vi "Get SMO Name.vi"(8 "error in (no error)":errorcluster, 11 "Instrument.FrameworkTemplate":refnum<class "Instrument.Temperhum.lvclass">) -> (0 "error out":errorcluster, 2 "SMO Name":string, 3 "Instrument.FrameworkTemplate out":refnum<class "Instrument.Temperhum.lvclass">)   [LabVIEW 2019, in "Instrument.Temperhum.lvclass"]
uses:
  Instrument.Temperhum.lvclass
  <userlib>/LevyLab/Instrument Framework/Instrument Types/VSource/Instrument.VSource.lvclass
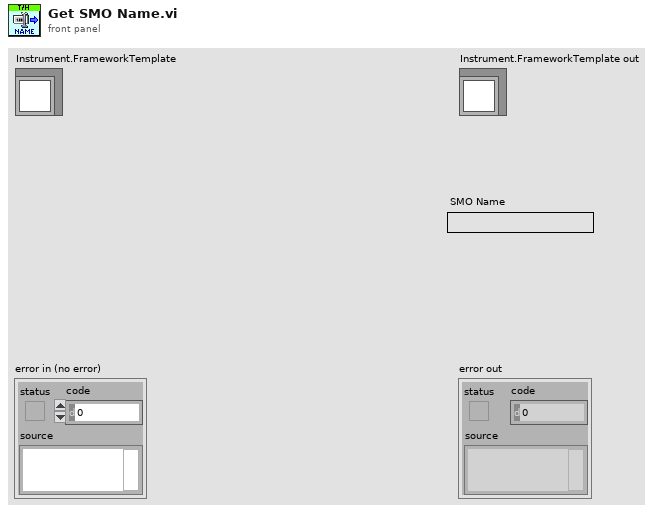
[diagram p1: front panel]
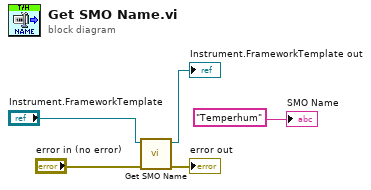
[diagram p0: block diagram]
diagram:
  n1 = call-parent "Get SMO Name.vi"("error in (no error)"="error in (no error)", "Instrument in"="Instrument.FrameworkTemplate") -> ("error out"=→"error out":errorcluster, "Instrument out"=→"Instrument.FrameworkTemplate out":refnum<class "Instrument.Temperhum.lvclass">)  [unwired: 7 in, 1 out]
  "SMO Name" <- "Temperhum" ("SMO Name")
